vi "ADC INL_sweep_triangle_ExtRef.vi"(8 "error in (no error)":errorcluster, 9 "Sequence parameters":string[][](array[string])=[["Min limit", "Max limit", "Register sheet file", "Register Sheet"], ["", "", "CC2600.xls", "TX_BLE;Trim"], ["Reg write (addr;value)", "Operating frequency [Hz]", "", ""], ["NA", "2.44G", "", ""]], 10 "Run type":i32, 11 "Method parameters":T3={"Dev"={"Do not disturb DUT"=FALSE, "XOSC"=32000000.0, "Board type"="", "EM"="", "Configure tempboard"=TRUE, "Device specific info"=[], "Generic Object"=refnum}, "Method"={"Run type"=1, "Test name"="Current LPM2 4", "Comment"="", "Results folder"="", "AFC"=enum."Off", "Method name"="Current LPM2 4", "Method results"={"Excel brief report"=FALSE, "Spotfire report"=FALSE, "Starfish report"=FALSE}, "Operator"="", "Reference time"=timestamp(0 s since 1904-01-01), "AFC delay"=0.0, "Initialization"=enum."Enabled", "MD5 Sum"="", "HW addon board"=enum."None", "AFC Regsheet"="", "AFC Regfile"=path "", "dummy"=0.0}, "Inst"={"Instr"={"PS1"={"Name"="", "GPIB address"="", "VISA session"=""}, "PS2"={"Name"="", "GPIB address"="", "VISA session"=""}, "TC1"={"Name"="", "GPIB address"="", "VISA session"=""}, "TC2"={"Name"="", "GPIB address"="", "VISA session"=""}, "SA1"={"Name"="", "GPIB address"="", "VISA session"=""}, "SA2"={"Name"="", "GPIB address"="", "VISA session"=""}, "SG1"={"Name"="", "GPIB address"="", "VISA session"=""}, "SG2"={"Name"="", "GPIB address"="", "VISA session"=""}, "SG3"={"Name"="", "GPIB address"="", "VISA session"=""}, "MI1"={"Name"="", "GPIB address"="", "VISA session"=""}, "MI2"={"Name"="", "GPIB address"="", "VISA session"=""}, "SW SA"={"Name"="", "Controller addr"=""}, "SW SG"={"Name"="", "Controller addr"=""}, "MI3"={"Name"="", "GPIB address"="", "VISA session"=""}}, "Switchbox"={"RF Path"=0, "Cal compensation"=enum."TX", "Switchbox gain mode"="", "State"=enum."TX"}, "Instr to control (i.e. SA1)"="Default", "Intrument info string"=""}, "Sequence parameters"=[["Weight", "Min Limit", "Max Limit", "Register Sheet", "", "", "", "", "", "", "", "", ""], ["Vital", "", "1", "LPM2", "", "", "", "", "", "", "", "", ""], ["Resolution", "Reg write (addr;value)", "Chip mode", "Range", "", "", "", "", "", "", "", "", ""], ["u", "NA", "", "auto", "", "", "", "", "", "", "", "", ""]], "Cond"={"Temp logged"=25.0, "VDD1_PS1_6V"=-999.0, "VDD2_PS1_25V"=-999.0, "VDD4_PS2_25V"=-999.0, "VDD3_PS2_6V"=-999.0}, "Meas config"={"X-axis inner loop index"=32000000, "Y-axis outer loop index"=32000000, "X-axis"=[], "Y-axis"=[], "X-axis array req size"=32000000, "Y-axis array req size"=32000000, "Param description"=[], "Use meas clust for reporting"=FALSE, "Parameter index (page)"=0, "X-axis name"="", "Y-axis name"=""}} {"Cond"."VDD3_PS2_6V" format="%.3f"; "Cond"."VDD4_PS2_25V" format="%.3f"; "Cond"."VDD2_PS1_25V" format="%.3f"; "Cond"."VDD1_PS1_6V" format="%.3f"; "Method"."dummy" format="%.1p"; "Method"."AFC delay" format="%.1p"; "Dev"."XOSC" format="%.3p"}) -> (0 "error out":errorcluster, 1 "End method error":T2, 2 "Short Results":string[](array[string])=["0.00", "0.00", "0.00", "0.00"], 3 "Result summary":string[][](array[string])=[["Critical", "Output Power@2405 MHz", "-3", "4", "dBm"], ["Critical", "Output Power@2410 MHz", "-3", "4", "dBm"]])   [LabVIEW 2019]
doc: "[AutoDocStart]Performs crystal accuracy measurements. Measures the offset from ideal frequency. Primarily used for tuning XOSC capacitors and verifying XOSC trims.\n\nSweeping parameters: operating frequency, OSC override value and VDDR level\n\nResults: Offset frequency in ppm[AutoDocEnd]"
uses:
  User Lib/Utilities/Cluster definitions/Method input.ctl
  User Lib/Utilities/Cluster definitions/Device specific info.ctl
  User Lib/Utilities/Controls/Automatic Frequency Compensation types.ctl
  User Lib/Utilities/Controls/Method Reports.ctl
  User Lib/Utilities/Cluster definitions/Method Initialization.ctl
  User Lib/Utilities/Controls/HW addon boards.ctl
  User Lib/Utilities/Cluster definitions/Instr clust.ctl
  User Lib/Utilities/Switchbox control/SwitchBox_State._ENUMctl.ctl
  User Lib/Utilities/Cluster definitions/End method error cluster.ctl
  User Lib/Utilities/Cluster definitions/DUT vdd control.ctl
  User Lib/Utilities/Cluster definitions/DUT VDD4.ctl
  User Lib/Utilities/Cluster definitions/DUT VDD3.ctl
  User Lib/Utilities/Cluster definitions/DUT VDD2.ctl
  User Lib/Utilities/Cluster definitions/DUT VDD1.ctl
  3a26386c-adf8-4bfd-9313-23d3b8777f38.vi
  4f05bcd1-6631-4ae4-b1ef-783b9f5d7cd6.vi
  0cf306e2-4f11-4798-8496-813b42596c0a.vi
panel:
  in  "Tab Control":T1(tab)
  # "°C"
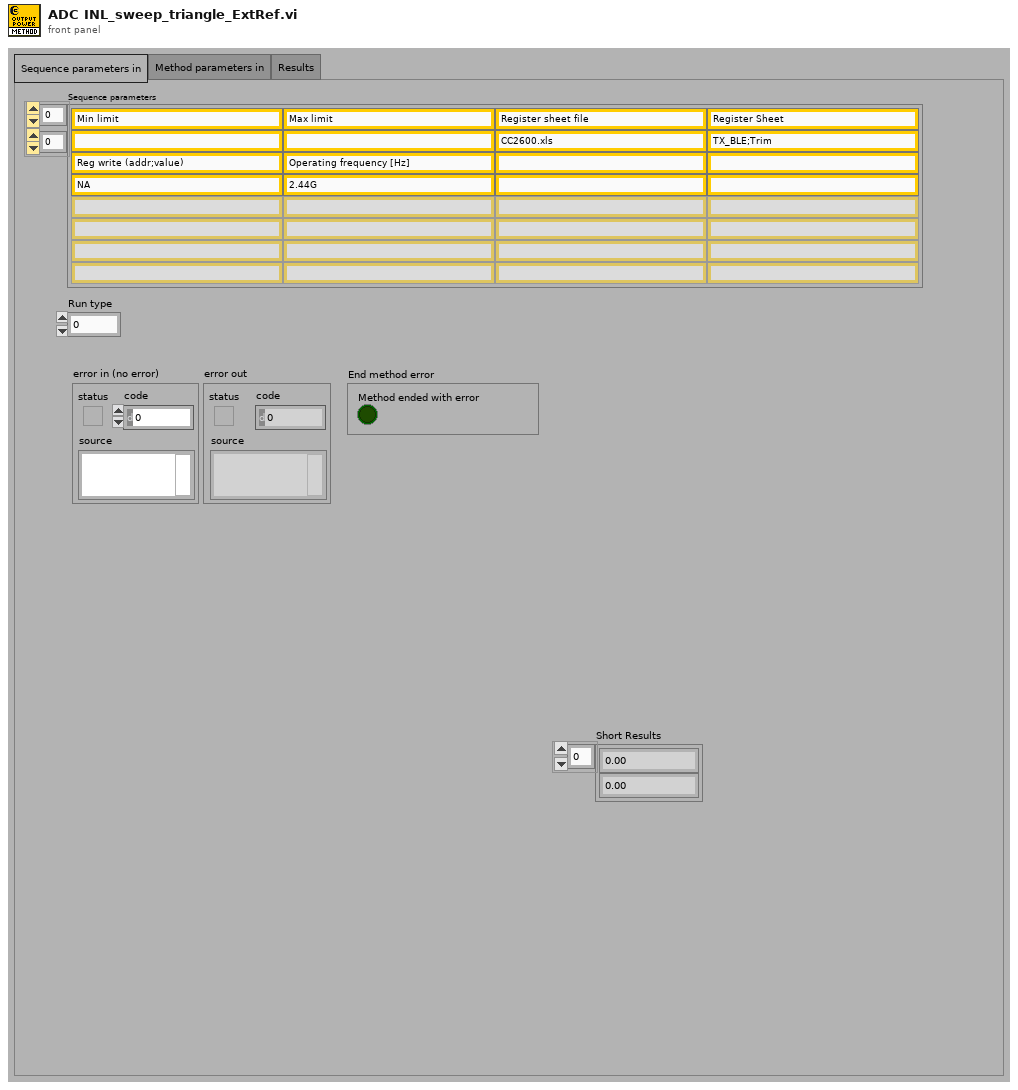
[diagram p1: front panel]
types:
  T1 = enum32{"Sequence parameters in", "Method parameters in", "Results"}
  T2 = typedef "End method error cluster.ctl" = cluster{"Method ended with error":bool}
  T3 = typedef "Method input.ctl" = cluster{"Dev":cluster{"Do not disturb DUT":bool, "XOSC":dbl, "Board type":string, "EM":string, "Configure tempboard":bool, "Device specific info":T4[], "Generic Object":refnum<class>}, "Method":cluster{"Run type":i32, "Test name":string, "Comment":string, "Results folder":string, "AFC":T5, "Method name":string, "Method results":T6, "Operator":string, "Reference time":timestamp, "AFC delay":dbl, "Initialization":T7, "MD5 Sum":string, "HW addon board":T8, "AFC Regsheet":string, "AFC Regfile":path, "dummy":dbl}, "Inst":T9, "Sequence parameters":string[][], "Cond":cluster{"Temp logged":dbl, "VDD1_PS1_6V":dbl, "VDD2_PS1_25V":dbl, "VDD4_PS2_25V":dbl, "VDD3_PS2_6V":dbl}, "Meas config":cluster{"X-axis inner loop index":i32, "Y-axis outer loop index":i32, "X-axis":string[], "Y-axis":string[], "X-axis array req size":i32, "Y-axis array req size":i32, "Param description":string[][], "Use meas clust for reporting":bool, "Parameter index (page)":i32, "X-axis name":string, "Y-axis name":string}}
  T4 = typedef "Device specific info.ctl" = cluster{"EM number":u8, "IP address":string, "Enabled":bool, "Slot no":u8, "RF path":u8, "EM name":string, "Wafer info":string, "AFC frequency ppm":dbl, "Register writes":string[][], "Meas data":string[][][], "Device comment":string}
  T5 = typedef "Automatic Frequency Compensation types.ctl" = enum16{"Off", "Compensate Instrument frequency", "Compensate DUT frequency", "Predictive - Compensate Instrument frequency", "Predictive - Compensate DUT frequency", "Do not skip re-init - Compensate Instrument frequency", "Do not skip re-init - Compensate DUT frequency"}
  T6 = typedef "Method Reports.ctl" = cluster{"Excel brief report":bool, "Spotfire report":bool, "Starfish report":bool}
  T7 = typedef "Method Initialization.ctl" = enum16{"Enabled", "Skip Instr and Device Init", "Enabled with Separate Flash", "Set PS, Device Init and Skip Instr Init", "Skip Device Init"}
  T8 = typedef "HW addon boards.ctl" = enum16{"None", "Current meas 5EM", "Stresstest 10EM"}
  T9 = typedef "Instr clust.ctl" = cluster{"Instr":cluster{"PS1":cluster{"Name":string, "GPIB address":string, "VISA session":refnum<visa-resource-name>}, "PS2":cluster{"Name":string, "GPIB address":string, "VISA session":refnum<visa-resource-name>}, "TC1":cluster{"Name":string, "GPIB address":string, "VISA session":refnum<visa-resource-name>}, "TC2":cluster{"Name":string, "GPIB address":string, "VISA session":refnum<visa-resource-name>}, "SA1":cluster{"Name":string, "GPIB address":string, "VISA session":refnum<visa-resource-name>}, "SA2":cluster{"Name":string, "GPIB address":string, "VISA session":refnum<visa-resource-name>}, "SG1":cluster{"Name":string, "GPIB address":string, "VISA session":refnum<visa-resource-name>}, "SG2":cluster{"Name":string, "GPIB address":string, "VISA session":refnum<visa-resource-name>}, "SG3":cluster{"Name":string, "GPIB address":string, "VISA session":refnum<visa-resource-name>}, "MI1":cluster{"Name":string, "GPIB address":string, "VISA session":refnum<visa-resource-name>}, "MI2":cluster{"Name":string, "GPIB address":string, "VISA session":refnum<visa-resource-name>}, "SW SA":cluster{"Name":string, "Controller addr":string}, "SW SG":cluster{"Name":string, "Controller addr":string}, "MI3":cluster{"Name":string, "GPIB address":string, "VISA session":refnum<visa-resource-name>}}, "Switchbox":cluster{"RF Path":i32, "Cal compensation":enum16{"TX", "RX", "Interferer", "No compensation", "Interferer2"}, "Switchbox gain mode":string, "State":T10}, "Instr to control (i.e. SA1)":string, "Intrument info string":string}
  T10 = typedef "SwitchBox_State._ENUMctl.ctl" = enum16{"TX", "RX", "SP:TX", "SP:RX", "SW:TX", "SW:RX"}
  T11 = typedef "DUT vdd control.ctl" = cluster{"VDD4 config":T12, "VDD3 config":T13, "VDD2 config":T14, "VDD1 config":T15}
  T12 = typedef "DUT VDD4.ctl" = u16
  T13 = typedef "DUT VDD3.ctl" = u16
  T14 = typedef "DUT VDD2.ctl" = u16
  T15 = typedef "DUT VDD1.ctl" = u16
  T16 = enum32{"NI Card Settings", "Memory Read Setting", "DC Capture", "ADC Ramp", "ADC Sine", "SNR", "Cap Calibration"}
  T17 = enum32{"Read from Memory", "Read .dat file", "NI Card Capture", "None"}
  T18 = cluster{"Path to Save plot":path, "Path to Raw Data plot":path}
  T19 = cluster{"Save INL/DNL Plot(Ramp)":bool, "Save SNR Plot":bool, "Save INL/DNL Plot(Sine)":bool, "Save INL/DNL Raw Data(Ramp)":bool, "Save SNR Raw Data":bool, "Save INL/DNL Raw Data(Sine)":bool, "Save DC Raw data":bool, "Save  Raw Data(Sine)":bool}
  T20 = cluster{"Min INL":dbl, "Max INL":dbl, "Min DNL":dbl, "Max DNL":dbl, "INL Range":dbl, "DNL Range":dbl, "Avg Hits/Code":dbl}
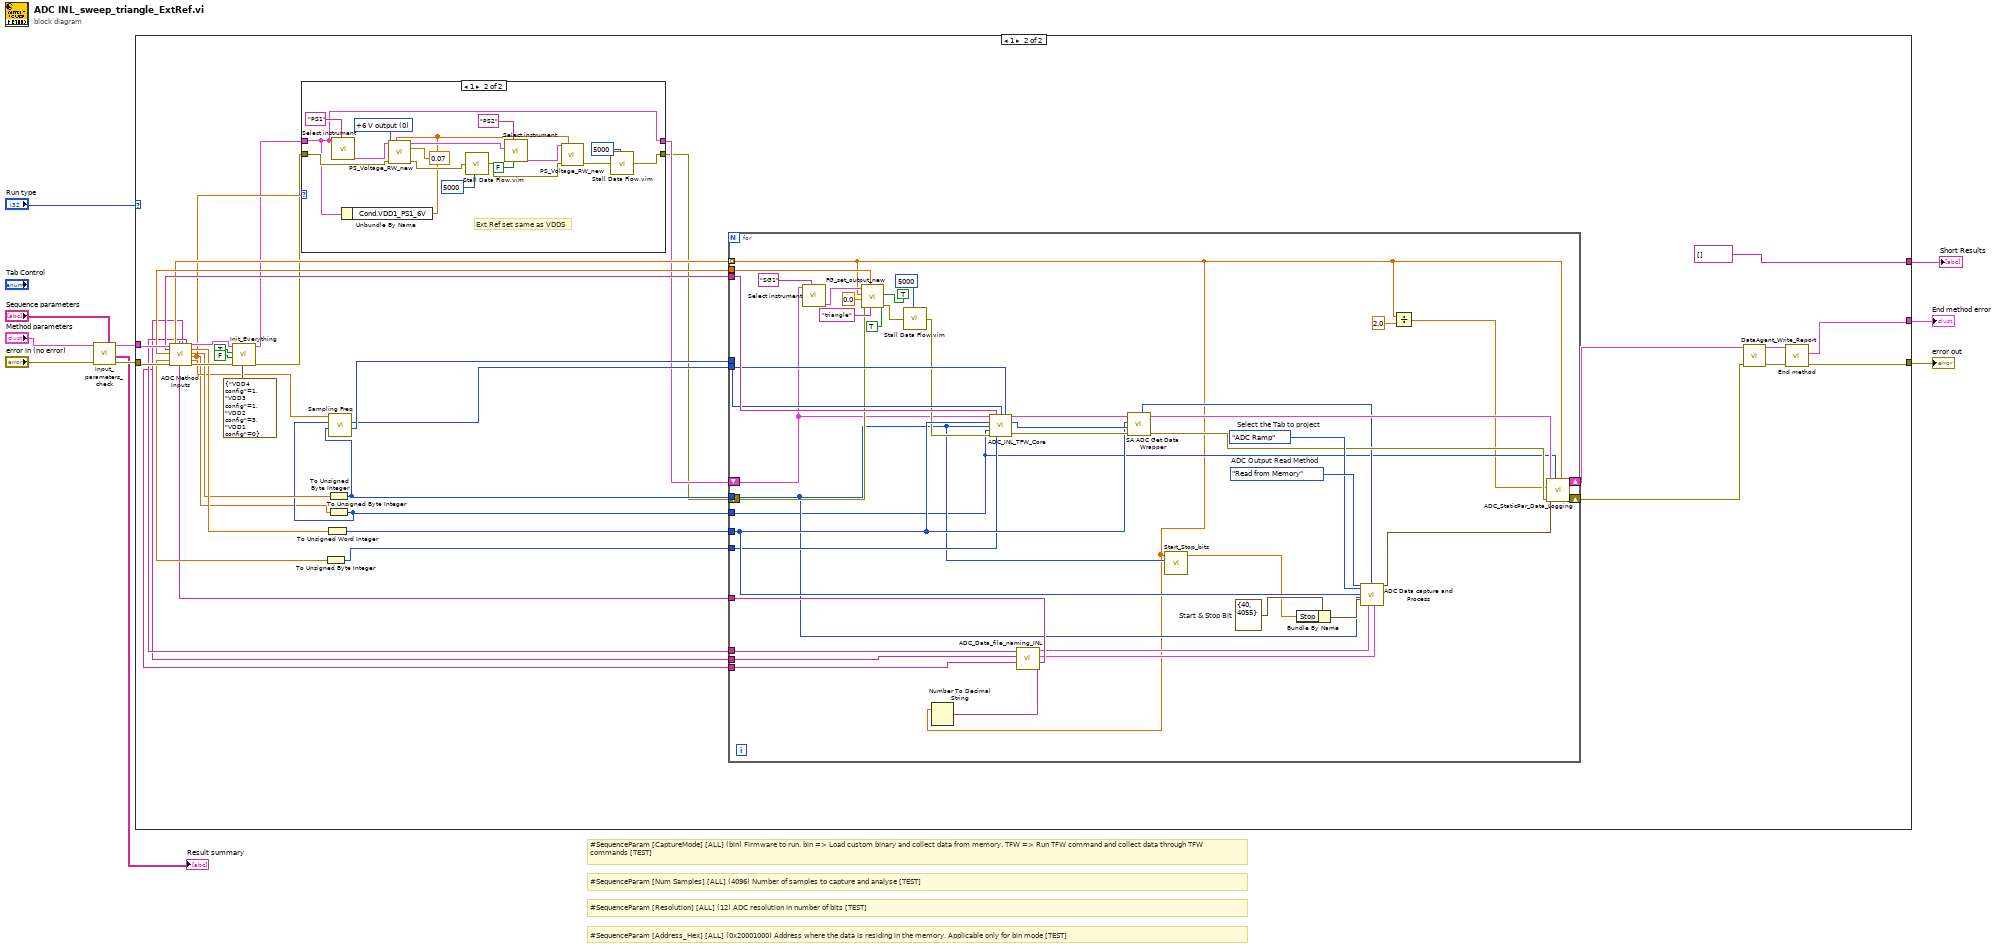
[diagram p0: block diagram]
diagram:
  # "#SequenceParam [Num Samples] [ALL] (4096) Number of samples to capture and analyse [TEST]"
  # "#SequenceParam [CaptureMode] [ALL] (bin) Firmware to run. bin => Load custom binary and collect data from memory. TFW => Run TFW command and collect data through TFW commands [TEST]"
  # "#SequenceParam [Address_Hex] [ALL] (0x20001000) Address where the data is residing in the memory. Applicable only for bin mode [TEST]"
  # "#SequenceParam [Resolution] [ALL] (12) ADC resolution in number of bits [TEST]"
  n1 = call "Input_parameters_check.vi"("Sequence parameters"="Sequence parameters", "error in"="error in (no error)", "Method cluster in"="Method parameters") -> ("error out"=w9:errorcluster, "Result summary"=→"Result summary":string[][], "Method cluster out"=w5:T3)  [unwired: 6 in]
  n2 = case shown="1" "Run type" {
    tunnel: w9 -> [w11 w36]
    tunnel: [w11 w47] -> w10
    tunnel: w5 -> [_ w37]
    tunnel: [_ w46] -> w4
    tunnel: [_ string[] []] -> w1
    frame 0, Default {
      # "Run type 0 is only for formatting the result summary"
    }
    frame 1 {
      n3 = call "ADC Method Inputs.vi"("Method cluster in"=w37, "error in (no error)"=w36) -> ("Capture Mode"=w26:string, "Signal Freq"=w22:dbl, "ADC Chnl No."=w30:dbl, "Input Voltage"=w21:dbl[], "Sampling Freq String"=w18:string, "Chnl No. string"=w17:string, "Resolution String"=w19:string, "Voltage Ref String"=w20:string, "Method cluster out"=w34:T3, "Num Samples"=w33:dbl, "Resolution"=w32:dbl, "Voltage Ref"=w16:dbl, "Sampling Freq"=w31:dbl, "error out"=w35:errorcluster)  [unwired: 3 in, 1 out]
      n4 = call "Init_Everything.vi"("VDD config"=T11 {"VDD4 config"=1, "VDD3 config"=1, "VDD2 config"=3, "VDD1 config"=0}, "error in"=w35, "Support current measurement?"=FALSE, "Override VDD Config"=TRUE, "Method cluster In"=w34) -> ("error out"=w13:errorcluster, "Method cluster out"=w15:T3)  [unwired: 3 in, 2 out]
      n5 = case shown="1" w16 {
        tunnel: w15 -> [w49 w53]
        tunnel: [w49 w53] -> w14
        tunnel: w13 -> [w48 w61]
        tunnel: [w48 w51] -> w12
        frame 0, 2, 3, Default {
        }
        frame 1 {
          w64 = u16 0 items=["+6 V output", "+25 V output", "-25 V output", "ALL TERM"] ("Output Terminals")
          # "Ext Ref set same as VDDS"
          n6 = call "Select instrument.vi"("Instr.Instr to control (i.e. SA1)"="PS1", "Method cluster in"=w53) -> ("Instr out"=w65:T9)  [unwired: 7 in, 2 out]
          n7 = Unbundle By Name(w53) -> ("Cond.VDD1_PS1_6V"=w55:dbl)
          n8 = call "PS_Voltage_RW_new.vi"("InstrCluster in"=w65, "Set Voltage"=w55, "Current(0)"=0.07, "Output Terminals"=w64, "error in (no error)"=w61) -> ("InstrCluster out"=w59:T9, "error out"=w62:errorcluster)  [unwired: 8 in, 1 out]
          n9 = call "Stall Data Flow.vim"("value in"=w62, "milliseconds to wait"=u32 5000) -> ("value out"=w54:errorcluster)  [unwired: 1 out]
          n10 = call "Select instrument.vi"("Method cluster (T) / Instr cluster (F)"=FALSE, "Instr.Instr to control (i.e. SA1)"="PS2", "Instr in"=w59) -> ("Instr out"=w56:T9)  [unwired: 6 in, 2 out]
          n11 = call "PS_Voltage_RW_new.vi"("InstrCluster in"=w56, "Set Voltage"=w55, "error in (no error)"=w54) -> ("error out"=w52:errorcluster)  [unwired: 10 in, 2 out]
          n12 = call "Stall Data Flow.vim"("value in"=w52, "milliseconds to wait"=u32 5000) -> ("value out"=w51:errorcluster)  [unwired: 1 out]
        }
      }
      n13 = To Unsigned Byte Integer(number=w30) -> (unsigned 8bit integer=w27:u8)
      n14 = To Unsigned Word Integer(number=w33) -> (unsigned 16bit integer=w29:u16)
      n15 = To Unsigned Byte Integer(number=w32) -> (unsigned 8bit integer=w28:u8)
      n16 = To Unsigned Byte Integer(number=w16) -> (unsigned 8bit integer=w23:u8)
      n17 = call "Sampling Freq.vi"("Resolution"=w28, "Voltage Ref"=w23, "Sampling Freq"=w31) -> ("LGPT Count"=w25:u16, "SCOMP"=w24:u16)  [unwired: 7 in]
      n18 = for {
        tunnel: w29 -> [w99]
        tunnel: w28 -> [w72]
        tunnel: w23 -> [w70]
        tunnel: w27 -> [w98]
        tunnel: w26 -> [w97]
        tunnel: w25 -> [w96]
        tunnel: w24 -> [w95]
        shift-right: [w104] -> w41
        shift-left: w14 -> [w89]
        shift-right: [w103] -> w40
        shift-left: w12 -> [w92]
        tunnel: w21 -> [w69] mode=indexing
        tunnel: w22 -> [w86]
        tunnel: w20 -> [w81]
        tunnel: w19 -> [w83]
        tunnel: w18 -> [w82]
        tunnel: w17 -> [w80]
        w76 = cluster{"Start":i32, "Stop":i32} {"Start"=40, "Stop"=4055}  # Start & Stop Bit
        w108 = T16."ADC Ramp"  # Select the Tab to project
        w109 = T17."Read from Memory"  # ADC Output Read Method
        n19 = call "Select instrument.vi"("Instr.Instr to control (i.e. SA1)"="SG1", "Method cluster in"=w89) -> ("Instr out"=w94:T9)  [unwired: 7 in, 2 out]
        n20 = call "FG_set_output_new.vi"("High impedance (T)"=TRUE, "Enable Output?"=TRUE, "Function (DC, Sine, Square, Triangle, Ramp up, Ramp down, Pulse)"="triangle", "Frequency [Hz]"=w86, "error in"=w92, "Low voltage"=0.0, "High voltage (or DC)"=w69, "InstrCluster in"=w94) -> ("error out"=w91:errorcluster)  [unwired: 2 in, 1 out]
        n21 = call "Stall Data Flow.vim"("value in"=w91, "milliseconds to wait"=u32 5000) -> ("value out"=w90:errorcluster)  [unwired: 1 out]
        n22 = Number To Decimal String(number=w69) -> (decimal integer string=w71:string)  [unwired: 1 in]
        n23 = call "ADC_INL_TFW_Core.vi"("Method cluster in"=w89, "Capture Mode"=w97, "LGPT Count"=w96, "SCOMP"=w95, "No. Samples"=w99, "Resolution"=w72, "Voltage Ref"=w70, "error in"=w90, "ADC Chnl No."=w98) -> ("Method cluster out"=w74:T3, "ResPar[0] Data Address"=w100:u32, "error out"=w101:errorcluster)  [unwired: 3 in, 1 out]
        n24 = call "ADC_Data_file_naming_INL.vi"("Amplitude (Vpp)"=w71, "ADC Chn. No"=w80, "Sampling Freq String"=w82, "Resolution String"=w83, "Voltage Ref String"=w81) -> ("path to save"=w78:T18, "Save data"=w79:T19)  [unwired: 5 in]
        n25 = call "SA ADC Get Data Wrapper.vi"("error in"=w101, "Data Address"=w100, "Num Samples"=w99, "Method cluster in"=w74) -> ("error out"=w107:errorcluster, "output cluster"=w106:T3, "ADC samples"=w105:u32[])  [unwired: 2 in, 3 out]
        n26 = call "Start_Stop_bits.vi"("Resolution"=w72, "Input Amplitude"=w69) -> ("Stop Bit"=w73:dbl)  [unwired: 9 in]
        n27 = Bundle By Name(cluster=w76, "Stop"=w73) -> (w75:cluster{"Start":i32, "Stop":i32})
        n28 = call "ADC Data capture and Process.vi"("ADC Output Read Method"=w109, "Select the Tab to project"=w108, "No.of samples"=w99, "Resolution"=w72, "Start & Stop Bit"=w75, "Save data"=w79, "Input Waveform"=w105, "path to save"=w78) -> ("Static Parameters (Ramp)"=w102:T20)  [unwired: 14 in, 5 out]
        n29 = Divide(x=w69, y=2.0) -> (x/y=w67:dbl)
        n30 = call "ADC_StaticPar_Data_Logging.vi"("Offset (V)"=w67, "Amplitude (Vpp)"=w69, "Ref Voltage"=w70, "error in (no error)"=w107, "Static Parameters (Ramp)"=w102, "output cluster"=w106) -> ("error out"=w103:errorcluster, "Method cluster out"=w104:T3)  [unwired: 4 in]
      }
      n31 = call "DataAgent_Write_Report.vi"("error in (no error)"=w40, "Method cluster in"=w41) -> ("error out"=w44:errorcluster, "Method cluster out"=w43:T3)  [unwired: 8 in]
      n32 = call "End method.vi"("error in"=w44, "Method cluster in"=w43) -> ("error out"=w47:errorcluster, "End method error"=w46:T2)  [unwired: 7 in, 1 out]
    }
  }
  "error out" <- w10
  "End method error" <- w4
  "Short Results" <- w1
